vi "Tektronix AFG 3000 Series Amplitude Modulation.vi"() -> ()   [LabVIEW 2009, in "Tektronix AFG 3000 Series.lvlib"]
doc: "Demonstrates how to configure and generate an amplitude modulated waveform."
uses:
  Tektronix AFG 3000 Series.lvlib
  Public/Configure/Configure Modulation (Amplitude).vi
panel:
  in  "Modulation Depth (0 %)":dbl
  in  "Modulation Frequency (1000 Hz)":dbl[unit]=1000.0
  in  "Channel (0: Channel 1)":u16(ring) items=["Channel 1", "Channel 2"]
  in  "Modulation Waveform (0: Sine)":u16(ring) items=["Sine", "Square", "Triangle", "Ramp", "Down Ramp", "Noise"]
  in  "AM Source (0: Internal)":u16(ring) items=["Internal", "External"]
  in  "DC Offset (0.00 V)":dbl[unit]
  in  "Frequency (1000 Hz)":dbl[unit]=1000.0
  in  "Amplitude (1 Vpp)":dbl[unit]=1.0
  in  "Waveform Function (0: Sine)":u16(ring) items=["Sine", "Square", "Pulse", "Ramp", "Noise", "DC", "Sin(x)/x", "Gaussian", "Lorentz", "Exponential Rise", "Exponential Decay", "Haversine"]
  in  "VISA resource name":refnum<visa-resource-name>
  # "(c) 2006-2009 National Instruments.  ALL RIGHTS RESERVED."
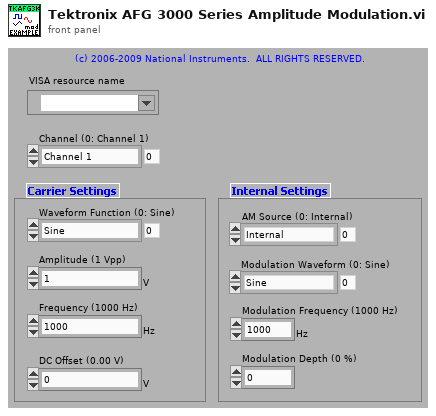
[diagram p1: front panel]
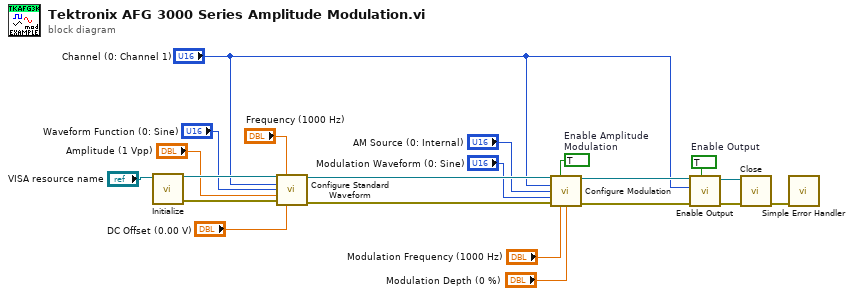
[diagram p0: block diagram]
diagram:
  w4 = TRUE  # Enable Output
  w7 = TRUE  # Enable Amplitude Modulation
  n1 = call "Initialize.vi"("VISA resource name"="VISA resource name") -> ("error out"=w12:errorcluster, "VISA resource name out"=w20:refnum<visa-resource-name>)  [unwired: 3 in, 6 out]
  n2 = call "Configure Standard Waveform.vi"("VISA resource name"=w20, "Frequency (1000 Hz)"="Frequency (1000 Hz)", "Channel (0: Channel 1)"="Channel (0: Channel 1)", "Waveform Function (0: Sine)"="Waveform Function (0: Sine)", "Amplitude (1 Vpp)"="Amplitude (1 Vpp)", "error in (no error)"=w12, "DC Offset (0.00 V)"="DC Offset (0.00 V)") -> ("VISA resource name out"=w19:refnum<visa-resource-name>, "error out"=w13:errorcluster)  [unwired: 1 in, 6 out]
  n3 = call-poly "Configure Modulation.vi"("VISA resource name"=w19, "Enable Amplitude Modulation (T: Enable)"=w7, "Channel (0: Channel 1)"="Channel (0: Channel 1)", "AM Source (0: Internal)"="AM Source (0: Internal)", "Modulation Waveform (0: Sine)"="Modulation Waveform (0: Sine)", "error in (no error)"=w13, "Modulation Frequency (1000 Hz)"="Modulation Frequency (1000 Hz)", "Modulation Depth (0 %)"="Modulation Depth (0 %)") -> ("VISA resource name out"=w18:refnum<visa-resource-name>, "error out"=w14:errorcluster)  [unwired: 1 in, 5 out]
  n4 = call "Enable Output.vi"("Enable Output (T: Enable)"=w4, "error in (no error)"=w14, "Channel (0: Channel 1)"="Channel (0: Channel 1)", "VISA resource name"=w18) -> ("error out"=w15:errorcluster, "VISA resource name out"=w17:refnum<visa-resource-name>)  [unwired: 6 out]
  n5 = call "Close.vi"("error in (no error)"=w15, "VISA resource name"=w17) -> ("error out"=w16:errorcluster)  [unwired: 9 out]
  n6 = call <vilib>:"Simple Error Handler.vi"("error in (no error)"=w16) -> ()  [unwired: 1 in, 8 out]
